vi "matematic operations.vi"() -> ()   [LabVIEW 2021]
panel:
  in  "tfin":dbl=5.0
  in  "fs":dbl=20.0
  out "it":i32=100
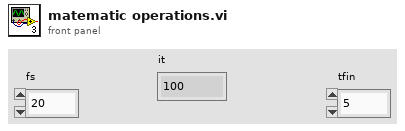
[diagram p1: front panel]
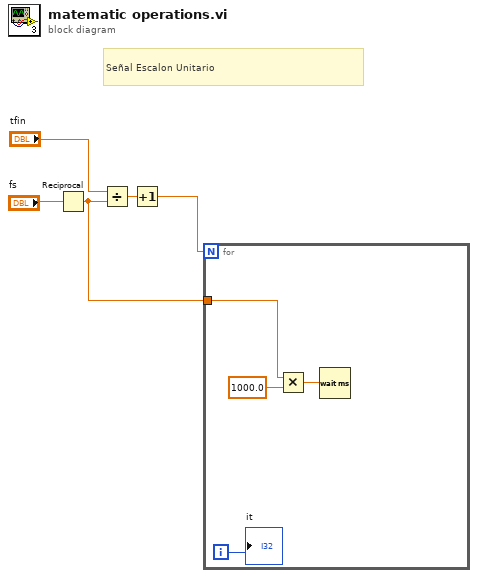
[diagram p0: block diagram]
diagram:
  # "Señal Escalon Unitario"
  n1 = Reciprocal(x="fs") -> (1/x=w1:dbl)
  n2 = Divide(x="tfin", y=w1) -> (x/y=w3:dbl)
  n3 = Increment(x=w3) -> (x+1=w2:dbl)
  n4 = for {
    N: w2 -> [_]
    tunnel: w1 -> [w6]
    i -> [w9]
    n5 = Multiply(x=w6, y=1000.0) -> (x*y=w8:dbl)
    n6 = Wait (ms)(milliseconds to wait=w8) -> ()  [unwired: 1 out]
    "it" <- w9
  }
